vi "isEmpty.vi"(8 "error in (no error)":errorcluster, 11 "MultiTree in":refnum<class "MultiTree.lvclass">) -> (0 "error out":errorcluster, 2 "empty":bool, 3 "MultiTree out":refnum<class "MultiTree.lvclass">)   [LabVIEW 2014, in "MultiTree.lvlib" / "MultiTree.lvclass"]
uses:
  <userlib>/AdvancedDataStructures/ClassBased/MultiTree/MultiTree.lvclass
  <userlib>/AdvancedDataStructures/ClassBased/MultiTree/MultiTree.lvclass/MultiTree.ctl
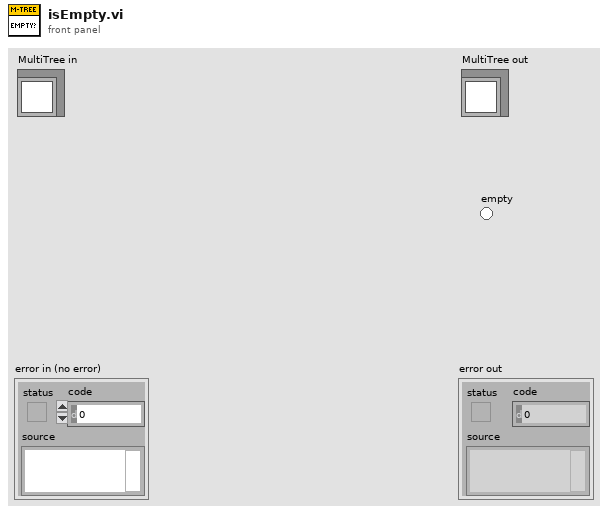
[diagram p1: front panel]
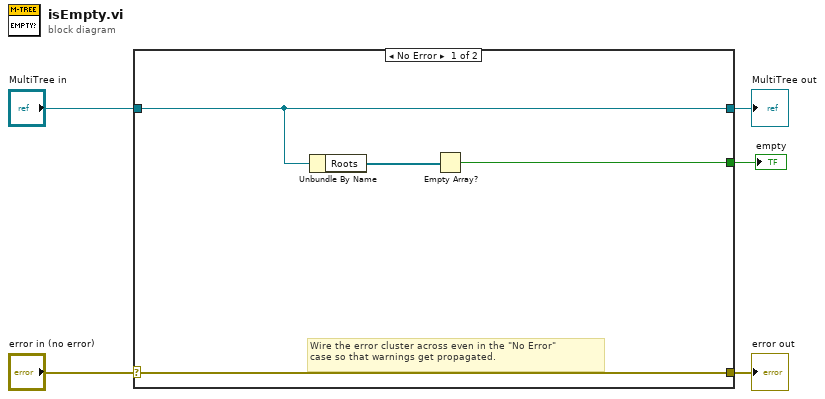
[diagram p0: block diagram]
diagram:
  n1 = case shown="No Error" "error in (no error)" {
    selector: "error in (no error)" -> [w9 w11]
    tunnel: [w9 w11] -> w4
    tunnel: [w8 w10] -> w2
    tunnel: "MultiTree in" -> [w8 w10]
    tunnel: [w6 _] -> w1
    frame No Error {
      # "Wire the error cluster across even in the \"No Error\"\ncase so that warnings get propagated."
      n2 = Unbundle By Name(w8) -> ("Roots"=w7:refnum<data-value>[])
      n3 = Empty Array?(array=w7) -> (empty?=w6:bool)
    }
    frame Error {
    }
  }
  "error out" <- w4
  "MultiTree out" <- w2
  "empty" <- w1
